vi "Auto 3.vi"(8 "Error In":errorcluster) -> (0 "Error Out":errorcluster)   [LabVIEW 2014]
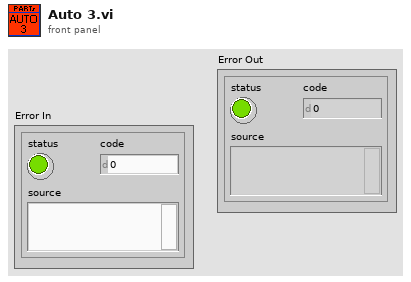
[diagram p1: front panel]
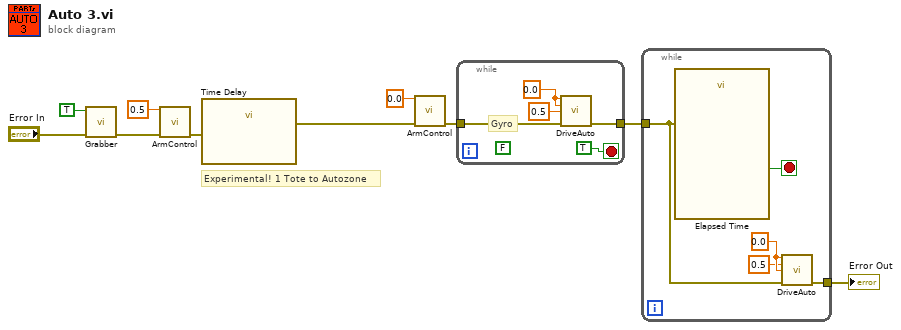
[diagram p0: block diagram]
diagram:
  # "Experimental! 1 Tote to Autozone"
  n1 = call "Grabber.vi"("Error In"="Error In", "Grabber Open/Close"=TRUE) -> ("Error Out"=w7:errorcluster)  [unwired: 9 in]
  n2 = call "ArmControl.vi"("Arm Value"=0.5, "Error In"=w7) -> ("Error Out"=w8:errorcluster)  [unwired: 13 in]
  n3 = call "Time Delay"("error in (no error)"=w8) -> ("error out"=w9:errorcluster)  [unwired: 10 in]
  n4 = call "ArmControl.vi"("Arm Value"=0.0, "Error In"=w9) -> ("Error Out"=w10:errorcluster)  [unwired: 13 in]
  n5 = while {
    tunnel: w10 -> [w15]
    tunnel: [w14] -> w5
    stop <- TRUE stop-if-true
    (unwired) FALSE ("Grabber Open/Close")
    w13 = 0.0 ("Arm Value")
    # "Gyro"
    n6 = call "DriveAuto.vi"("X In"=w13, "Y In"=w13, "R In"=0.5 ("X In"), "Error In"=w15) -> ("Error Out"=w14:errorcluster)  [unwired: 11 in]
  }
  n7 = while {
    tunnel: w5 -> [w16]
    tunnel: [w20] -> w4
    stop <- w17 stop-if-true
    w19 = 0.0 ("Arm Value")
    n8 = call "Elapsed Time"("error in (no error)"=w16) -> ("Time has Elapsed"=w17:bool)  [unwired: 11 in, 7 out]
    n9 = call "DriveAuto.vi"("X In"=w19, "Y In"=0.5 ("X In"), "R In"=w19, "Error In"=w16) -> ("Error Out"=w20:errorcluster)  [unwired: 11 in]
  }
  "Error Out" <- w4
